vi "Drive Core.vi"(0 "A Encoder BL":string="My Motor RefNum", 1 "Rotational Motor FR":string="My Motor RefNum", 2 "Rotational Motor FL":string="My Motor RefNum", 3 "Rotational Motor BR":string="My Motor RefNum", 4 "Rotational Motor BL":string="My Motor RefNum", 5 "Drive Motor FR":string="My Motor RefNum", 6 "A Encoder BR":string="My Motor RefNum", 7 "Drive Motor FL":string="My Motor RefNum", 8 "A Encoder FL":string="My Motor RefNum", 9 "Drive Motor BR":string="My Motor RefNum", 10 "A Encoder FR":string="My Motor RefNum", 11 "Drive Motor BL":string="My Motor RefNum") -> ()   [LabVIEW 2012]
uses:
  Global Variables.vi
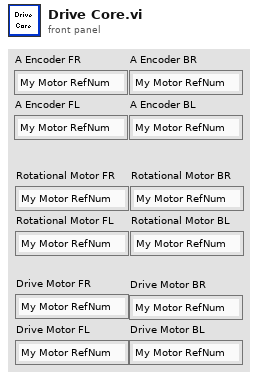
[diagram p1: front panel]
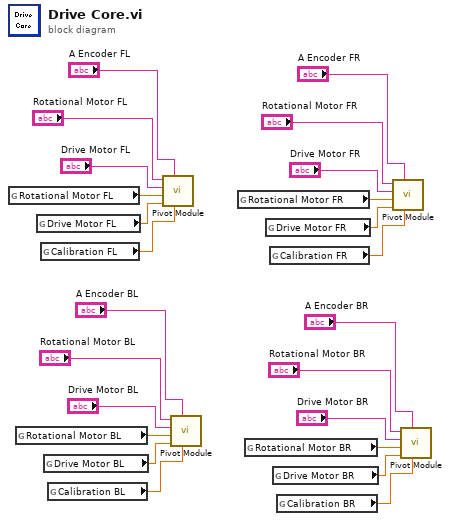
[diagram p0: block diagram]
diagram:
  n1 = global read "Global Variables.vi" "Rotational Motor FL"() -> (w3:dbl)
  n2 = global read "Global Variables.vi" "Rotational Motor BL"() -> (w1:dbl)
  n3 = global read "Global Variables.vi" "Drive Motor FL"() -> (w13:dbl)
  n4 = global read "Global Variables.vi" "Calibration FL"() -> (w4:dbl)
  n5 = global read "Global Variables.vi" "Drive Motor BL"() -> (w15:dbl)
  n6 = global read "Global Variables.vi" "Calibration BL"() -> (w6:dbl)
  n7 = call "Pivot Module.vi"("Calibration Angle"=w4, "Encoder Refnum"="A Encoder FL", "Motor Speed"=w13, "Motor Angle"=w3, "Drive Motor Refnum"="Drive Motor FL", "Rotational Motor Refnum"="Rotational Motor FL") -> ()  [unwired: 6 in]
  n8 = call "Pivot Module.vi"("Calibration Angle"=w6, "Encoder Refnum"="A Encoder BL", "Motor Speed"=w15, "Motor Angle"=w1, "Drive Motor Refnum"="Drive Motor BL", "Rotational Motor Refnum"="Rotational Motor BL") -> ()  [unwired: 6 in]
  n9 = global read "Global Variables.vi" "Rotational Motor FR"() -> (w21:dbl)
  n10 = global read "Global Variables.vi" "Rotational Motor BR"() -> (w2:dbl)
  n11 = global read "Global Variables.vi" "Drive Motor FR"() -> (w20:dbl)
  n12 = global read "Global Variables.vi" "Calibration FR"() -> (w19:dbl)
  n13 = global read "Global Variables.vi" "Drive Motor BR"() -> (w14:dbl)
  n14 = global read "Global Variables.vi" "Calibration BR"() -> (w5:dbl)
  n15 = call "Pivot Module.vi"("Calibration Angle"=w19, "Encoder Refnum"="A Encoder FR", "Motor Speed"=w20, "Motor Angle"=w21, "Drive Motor Refnum"="Drive Motor FR", "Rotational Motor Refnum"="Rotational Motor FR") -> ()  [unwired: 6 in]
  n16 = call "Pivot Module.vi"("Calibration Angle"=w5, "Encoder Refnum"="A Encoder BR", "Motor Speed"=w14, "Motor Angle"=w2, "Drive Motor Refnum"="Drive Motor BR", "Rotational Motor Refnum"="Rotational Motor BR") -> ()  [unwired: 6 in]
